vi "CAN_ReadErrInfo.vi"(8 "错误输入（无错误）":errorcluster, 11 "General_Input":T1={"DevType"=1, "DevIndex"=0, "CANIndex"=0} {"CANIndex" items=["0", "1"]; "DevType" items=["PCI5121"=1, "PCI9810"=2, "USBCAN1"=3, "USBCAN2"=4, "PCI9820"=5, "CAN232"=6, "PCI5110"=7, "CANLite(mini)"=8, "ISA9620"=9, "ISA5420"=10, "PC104CAN"=11, "CANETE"=12, "DNP9810"=13, "PCI9840B"=14, "PC104C2"=15, "PCI9820I"=16]}) -> (0 "错误输出":errorcluster, 3 "General_Output":T1={"DevType"=1, "DevIndex"=0, "CANIndex"=0} {"CANIndex" items=["0", "1"]; "DevType" items=["PCI5121"=1, "PCI9810"=2, "USBCAN1"=3, "USBCAN2"=4, "PCI9820"=5, "CAN232"=6, "PCI5110"=7, "CANLite(mini)"=8, "ISA9620"=9, "ISA5420"=10, "PC104CAN"=11, "CANETE"=12, "DNP9810"=13, "PCI9840B"=14, "PC104C2"=15, "PCI9820I"=16]})   [LabVIEW 2012]
panel:
  out "VCI_ERR_INFO":T2
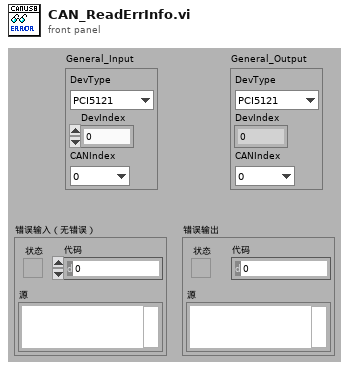
[diagram p1: front panel]
types:
  T1 = cluster{"DevType":u16, "DevIndex":u32, "CANIndex":u16}
  T2 = cluster{"ErrCode":u16, "Passive_ErrData 0":u8, "Passive_ErrData 1":u8, "Passive_ErrData 2":u8, "ArLost_ErrData":u8}
  T3 = cluster{"DevType":u32, "DevIndex":u32, "CANIndex":u32}
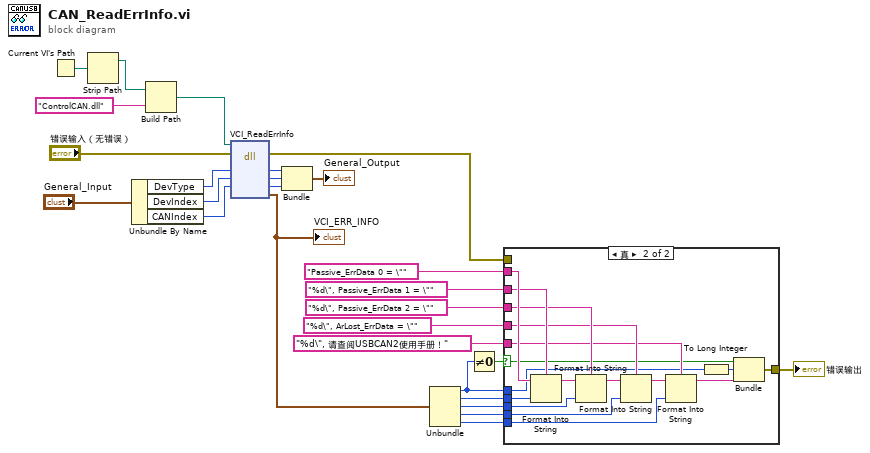
[diagram p0: block diagram]
diagram:
  n1 = Current VI's Path() -> (path=w10:path)
  n2 = Strip Path(path=w10) -> (stripped path=w11:path)  [unwired: 1 out]
  n3 = Unbundle By Name("General_Input") -> ("DevType"=w7:u16, "DevIndex"=w6:u32, "CANIndex"=w5:u16)
  n4 = Build Path(base path=w11, name or relative path="ControlCAN.dll" ("名称或相对路径")) -> (appended path=w8:path)
  n5 = dll-call lib="?" fn="VCI_ReadErrInfo"(path in=w8, error in="错误输入（无错误）", "DevType"=w7, "DevIndex"=w6, "CANIndex"=w5) -> (error out=w13:errorcluster, "DevType"=w4:u32, "DevIndex"=w3:u32, "CANIndex"=w2:u32, "VCI_ERR_INFO"=w26:T2)  [unwired: 3 in, 1 out]
  "VCI_ERR_INFO" <- w26
  n6 = Bundle("DevType"=w4, "DevIndex"=w3, "CANIndex"=w2) -> (→"General_Output":T3)  [unwired: 1 in]
  n7 = Unbundle(w26) -> ("ErrCode"=w15:u16, "Passive_ErrData 0"=w24:u8, "Passive_ErrData 1"=w23:u8, "Passive_ErrData 2"=w22:u8, "ArLost_ErrData"=w21:u8)
  n8 = Not Equal To 0?(x=w15) -> (x != 0?=w25:bool)
  n9 = case shown="真" w25 {
    selector: w25 -> [_ w33]
    tunnel: w24 -> [_ w42]
    tunnel: w23 -> [_ w41]
    tunnel: w22 -> [_ w40]
    tunnel: w21 -> [_ w39]
    tunnel: "Passive_ErrData 0 = \"" -> [_ w38]
    tunnel: "%d\", Passive_ErrData 1 = \"" ("格式字符串") -> [_ w37]
    tunnel: "%d\", Passive_ErrData 2 = \"" -> [_ w36]
    tunnel: "%d\", ArLost_ErrData = \"" -> [_ w35]
    tunnel: "%d\", 请查阅USBCAN2使用手册！" -> [_ w34]
    tunnel: w15 -> [_ w32]
    tunnel: [w28 w29] -> w14
    tunnel: w13 -> [w28 _]
    frame False {
    }
    frame True {
      n10 = Format Into String(format string=w37, initial string=w38, w42) -> (resulting string=w45:string)  [unwired: 1 in, 1 out]
      n11 = Format Into String(format string=w36, initial string=w45, w41) -> (resulting string=w44:string)  [unwired: 1 in, 1 out]
      n12 = Format Into String(format string=w35, initial string=w44, w40) -> (resulting string=w43:string)  [unwired: 1 in, 1 out]
      n13 = Format Into String(format string=w34, initial string=w43, w39) -> (resulting string=w30:string)  [unwired: 1 in, 1 out]
      n14 = To Long Integer(number=w32) -> (32bit integer=w31:i32)
      n15 = Bundle(w33, w31, w30) -> (w29:errorcluster)  [unwired: 1 in]
    }
  }
  "错误输出" <- w14
